vi "Read UDP Read Connection.vi"(8 "error in (no error)":errorcluster, 11 "ENET_BS120x in":refnum<class "ENET_BS120x.lvclass">) -> (0 "error out":errorcluster, 2 "UDP Read Connection":refnum<k16>, 3 "ENET_BS120x out":refnum<class "ENET_BS120x.lvclass">)   [LabVIEW 2021, in "BS120x Driver.lvlib" / "ENET_BS120x.lvclass"]
uses:
  ENET_BS120x.lvclass
  ENET_BS120x.lvclass/ENET_BS120x.ctl
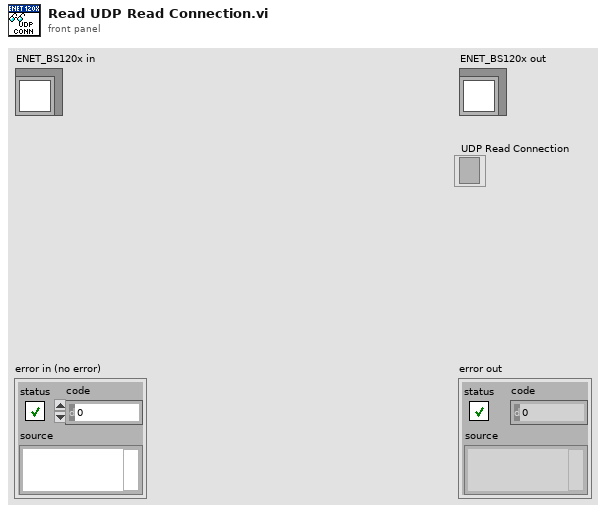
[diagram p1: front panel]
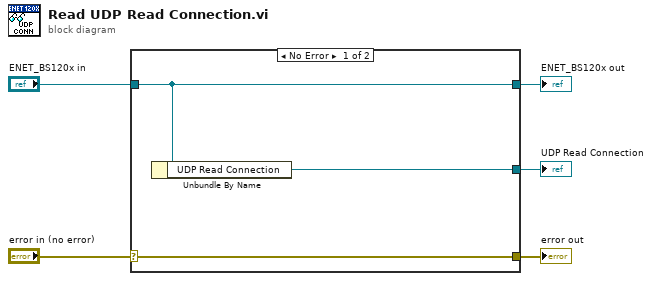
[diagram p0: block diagram]
diagram:
  n1 = case shown="No Error" "error in (no error)" {
    selector: "error in (no error)" -> [w8 w9]
    tunnel: [w8 w9] -> w4
    tunnel: [w7 w10] -> w2
    tunnel: "ENET_BS120x in" -> [w7 w10]
    tunnel: [w6 _] -> w1
    frame No Error {
      n2 = Unbundle By Name(w7) -> ("UDP Read Connection"=w6:refnum<k16>)
    }
    frame Error {
    }
  }
  "error out" <- w4
  "ENET_BS120x out" <- w2
  "UDP Read Connection" <- w1
